vi "Log Event.vi"(0 "Robot Notifications in":refnum<class "Robot Event Local Log.lvclass">, 1 "Program":string, 2 "data":variant, 5 "error in (no error)":errorcluster, 9 "Event Type":T1) -> (14 "Robot Notifications out":refnum<class "Robot Event Local Log.lvclass">, 19 "error out":errorcluster)   [LabVIEW 2019, in "Robot Event Local Log.lvclass"]
uses:
  Robot Event Local Log.lvclass
  C:/_Code/Development/Sub-Zero Functional Test/standard hardware/Universal Robots/UR LabVIEW Interface/Classes/Events/Robot Event/Robot Event.lvclass
  Robot Event/Event Type.ctl
  Robot Event Local Log.lvclass/Robot Event Local Log.ctl
  Robot Event/Robot Event.lvclass
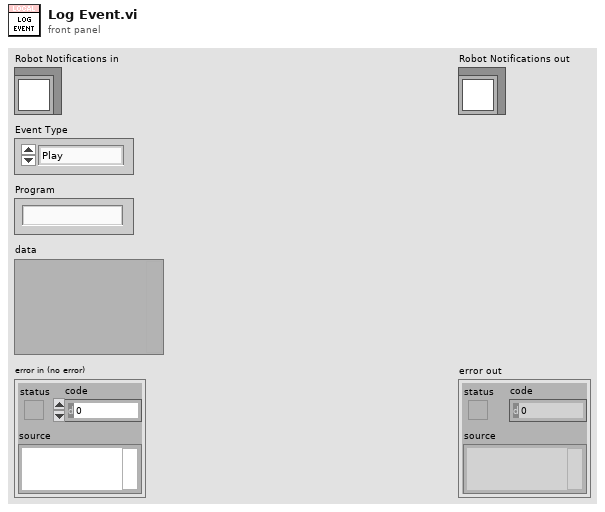
[diagram p1: front panel]
types:
  T1 = typedef "Robot Event.lvclass/Event Type.ctl" = enum16{"Play", "Error", "Fault", "Timeout", "Stopped", "Complete", "Fault - Program Resumed", "Fault - Program Aborted"}
  T2 = enum16{"open", "replace", "create", "open or create", "replace or create", "replace or create with confirmation"}
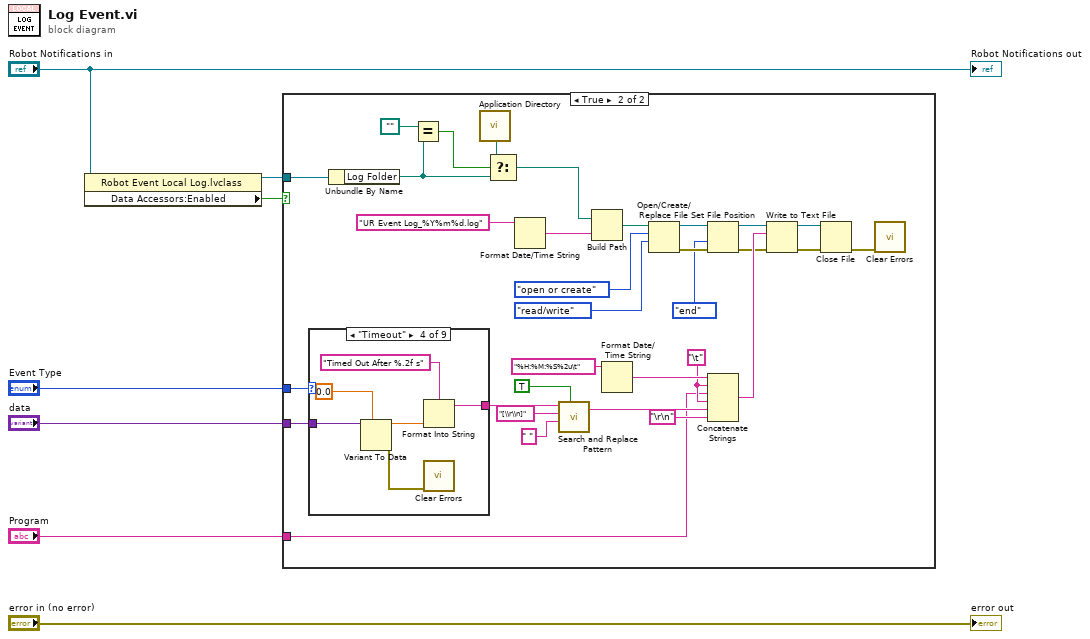
[diagram p0: block diagram]
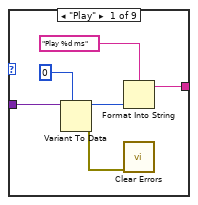
[diagram p3: hidden frame]
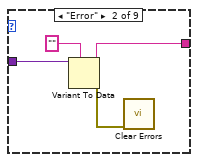
[diagram p4: hidden frame]
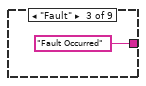
[diagram p5: hidden frame]
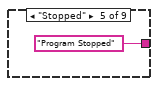
[diagram p6: hidden frame]
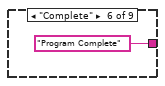
[diagram p7: hidden frame]
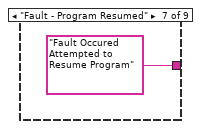
[diagram p8: hidden frame]
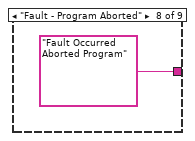
[diagram p9: hidden frame]
diagram:
  n1 = property class="Robot Event Local Log.lvclass"(reference="Robot Notifications in") -> (reference out=w1:refnum<class "Robot Event Local Log.lvclass">, "Data Accessors:Enabled"=w2:bool)  [unwired: 1 in, 1 out]
  n2 = case shown="True" w2 {
    tunnel: "Event Type" -> [_ w17]
    tunnel: "data" -> [_ w15]
    tunnel: "Program" -> [_ w14]
    tunnel: w1 -> [_ w13]
    frame False {
    }
    frame True {
      w19 = "\t" ("string")
      n3 = case shown="\"Timeout\"" w17 {
        tunnel: [w42 w46 "Fault Occurred" ("string") w53 "Program Stopped" ("string") "Program Complete" ("string") "Fault Occured Attempted to Resume Program" ("string") "Fault Occurred Aborted Program" ("string") _] -> w16
        tunnel: w15 -> [w45 w49 _ w56 _ _ _ _ _]
        frame "Play" {
          n4 = Variant To Data(type=0, Variant=w45) -> (data=w41:i32, error out=w43:errorcluster)  [unwired: 1 in]
          n5 = Format Into String(format string="Play %d ms", w41) -> (resulting string=w42:string)  [unwired: 2 in, 1 out]
          n6 = call <vilib>:"Clear Errors.vi"("error in (no error)"=w43) -> ()  [unwired: 5 in, 2 out]
        }
        frame "Error" {
          n7 = Variant To Data(type="", Variant=w49) -> (data=w46:string, error out=w48:errorcluster)  [unwired: 1 in]
          n8 = call <vilib>:"Clear Errors.vi"("error in (no error)"=w48) -> ()  [unwired: 5 in, 2 out]
        }
        frame "Fault" {
        }
        frame "Timeout" {
          n9 = Variant To Data(type=0.0, Variant=w56) -> (data=w52:dbl, error out=w54:errorcluster)  [unwired: 1 in]
          n10 = Format Into String(format string="Timed Out After %.2f s", w52) -> (resulting string=w53:string)  [unwired: 2 in, 1 out]
          n11 = call <vilib>:"Clear Errors.vi"("error in (no error)"=w54) -> ()  [unwired: 5 in, 2 out]
        }
        frame "Stopped" {
        }
        frame "Complete" {
        }
        frame "Fault - Program Resumed" {
        }
        frame "Fault - Program Aborted" {
        }
        frame Default {
        }
      }
      n12 = Unbundle By Name(w13) -> ("Log Folder"=w10:path)
      n13 = Equal?(x=path "", y=w10) -> (x = y?=w11:bool)
      n14 = call <vilib>:"Application Directory.vi"() -> ("Application Directory"=w8:path)
      n15 = Select(t=w8, s=w11, f=w10) -> (s? t:f=w9:path)
      n16 = Format Date/Time String(time format string (%c)="UR Event Log_%Y%m%d.log") -> (date/time string=w39:string)  [unwired: 2 in]
      n17 = call <vilib>:"Search and Replace Pattern.vi"("string"=w16, "regular expression (\"\")"="[\\r\\n]" ("regular expression (\"\")"), "replace string (\"\")"=" " ("replace string (\"\")"), "replace all? (F)"=TRUE) -> ("result string"=w30:string)  [unwired: 1 in, 1 out]
      n18 = Build Path(base path=w9, name or relative path=w39) -> (appended path=w38:path)
      n19 = Format Date/Time String(time format string (%c)="%H:%M:%S%2u\t") -> (date/time string=w35:string)  [unwired: 2 in]
      n20 = Open/Create/Replace File(file path (use dialog)=w38, operation (0:open)=T2."open or create", access (0:read/write)=enum16{"read/write", "read-only", "write-only"}."read/write") -> (refnum out=w23:refnum<file>, error out=w22:errorcluster)  [unwired: 3 in, 1 out]
      n21 = Set File Position(refnum=w23, from (0:start)=enum16{"start", "end", "current"}."end", error in=w22) -> (refnum out=w27:refnum<file>, error out=w26:errorcluster)  [unwired: 1 in]
      n22 = Concatenate Strings(w35, w19, w14, w19, w30, "\r\n") -> (w34:string)
      n23 = Write to Text File(file (use dialog)=w27, text=w34, error in=w26) -> (refnum out=w25:refnum<file>, error out=w24:errorcluster)  [unwired: 1 in, 1 out]
      n24 = Close File(refnum=w25, error in=w24) -> (error out=w18:errorcluster)  [unwired: 1 out]
      n25 = call <vilib>:"Clear Errors.vi"("error in (no error)"=w18) -> ()  [unwired: 5 in, 2 out]
    }
  }
  "error out" <- "error in (no error)"
  "Robot Notifications out" <- "Robot Notifications in"
